vi "hardware2.vi"() -> ()   [LabVIEW 2020]
uses:
  <vilib>/Platform/TimedLoop/XDataNode/timing_clust.ctl
  <vilib>/Platform/TimedLoop/XDataNode/nitl_modes.ctl
  <vilib>/Platform/TimedLoop/XDataNode/wakeup.ctl
  <vilib>/platform/TimedLoop/XDataNode/XDataNode.xnode
  <vilib>/Platform/TimedLoop/XDataNode/XDNodeRunTimeDep.lvlib
panel:
  out "latest notification":i32
  in  "stop":bool
  out "Numeric":i32
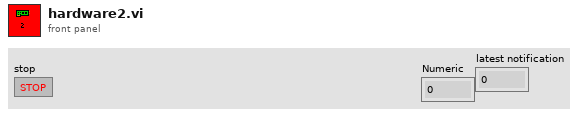
[diagram p1: front panel]
types:
  T1 = typedef "XDNodeRunTimeDep.lvlib/timing_clust.ctl" = cluster{"Expected End [f-1]":u64, "Actual End [f-1]":u64, "Finished Late? [f-1]":bool, "Expected End [i-1]":u64, "Actual End [i-1]":u64, "Finished Late? [i-1]":bool, "Expected Start [i]":u64, "Actual Start [i]":u64, "Expected Start [f]":u64, "Actual Start [f]":u64, "Source Name":string, "Structure Name":string, "Period":i64, "Deadline":i64, "Offset":i64, "Start":i64, "Priority":i32, "Timeout":i32, "Mode":T2, "Wakeup Reason":T3, "Error":errorcluster, "Source Type":string, "Secondary Source Type":string, "Global End Time":u64, "Global Start Time":u64, "Frame Duration":u64, "Iteration Duration":u64, "Assigned CPU":i32, "I/O Scan Engine Mode":u32}
  T2 = typedef "XDNodeRunTimeDep.lvlib/nitl_modes.ctl" = enum32{"No Change", "Process missed periods, maintain original phase", "Discard missed periods, maintain original phase", "Process missed periods, ignore original phase", "Discard missed periods, ignore original phase"}
  T3 = typedef "XDNodeRunTimeDep.lvlib/wakeup.ctl" = enum32{"Normal", "Aborted", "Asynchronous wakeup", "Timing source error", "Timed loop error", "Timeout"}
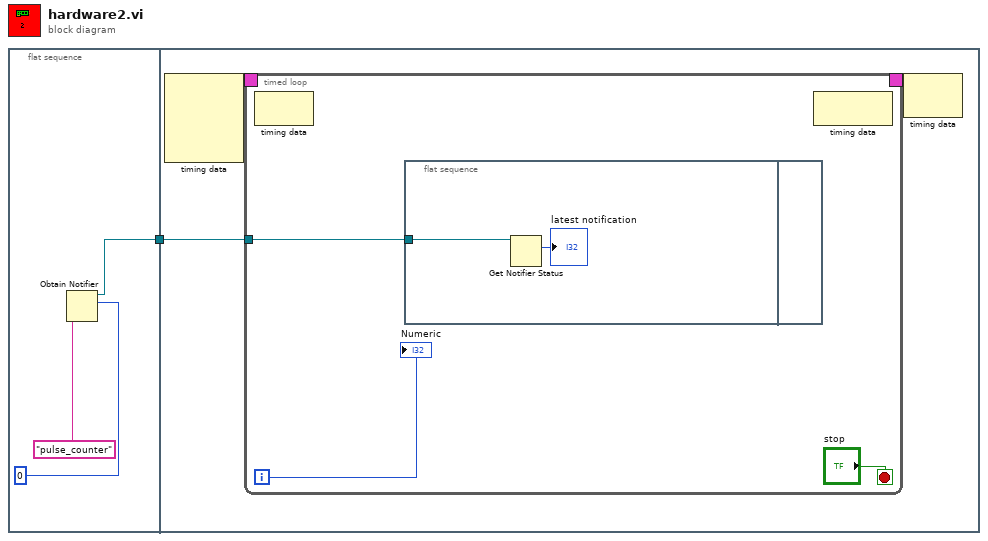
[diagram p0: block diagram]
diagram:
  n1 = flat-sequence {
    tunnel: [w2] -> w1
    tunnel: w1 -> [w5]
    frame #0 {
      n2 = Obtain Notifier(name (unnamed)="pulse_counter", notification data type=0) -> (notifier out=w2:refnum<notifier>)  [unwired: 2 in, 2 out]
    }
    frame #1 {
      n3 = node-c288() -> (w7:T1)  [unwired: 4 in]
      n4 = timed-loop {
        timing: w7 -> [_]
        timing-out: [_] -> w6
        tunnel: w5 -> [w8]
        i -> [w9]
        stop <- "stop" stop-if-true
        n5 = node-c288() -> ()  [unwired: 1 in, 1 out]
        n6 = flat-sequence {
          tunnel: w8 -> [w12]
          frame #0 {
            n7 = Get Notifier Status(notifier=w12) -> (current notification=→"latest notification":i32)  [unwired: 1 in, 4 out]
          }
          frame #1 {
          }
        }
        n8 = node-c288() -> ()  [unwired: 1 in, 1 out]
        "Numeric" <- w9
      }
      n9 = node-c288(w6) -> ()  [unwired: 1 out]
    }
  }
